vi "SRS830_GetXY.vi"(8 "error in (no error)":errorcluster, 11 "SRS 830":refnum<visa-resource-name>) -> (0 "error out (no error)":errorcluster, 1 "Y":dbl, 2 "X":dbl, 3 "SRS 830 Out":refnum<visa-resource-name>)   [LabVIEW 2014]
uses:
  Stanford Research 830/Stanford Research 830.lvlib
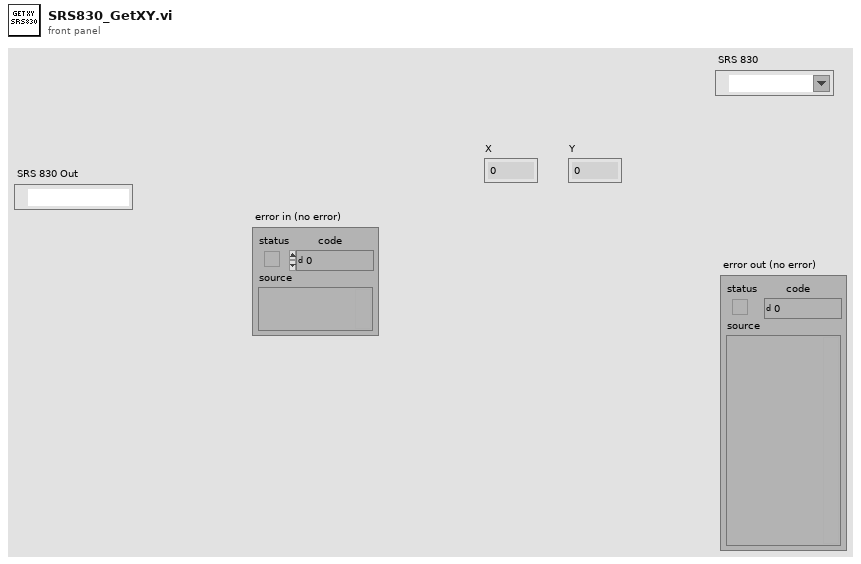
[diagram p1: front panel]
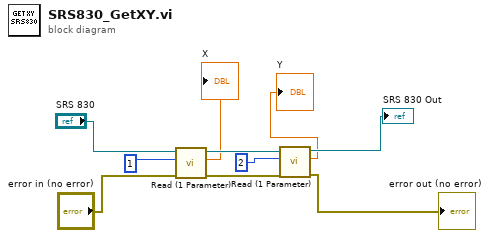
[diagram p0: block diagram]
diagram:
  n1 = call "Read (1 Parameter).vi"("error in (no error)"="error in (no error)", "Parameter (1: X)"=1, "VISA resource name"="SRS 830") -> ("error out"=w9:errorcluster, "Measurement"=→"X":dbl, "VISA resource name out"=w6:refnum<visa-resource-name>)  [unwired: 6 in]
  n2 = call "Read (1 Parameter).vi"("error in (no error)"=w9, "Parameter (1: X)"=2, "VISA resource name"=w6) -> ("error out"=→"error out (no error)":errorcluster, "Measurement"=→"Y":dbl, "VISA resource name out"=→"SRS 830 Out":refnum<visa-resource-name>)  [unwired: 6 in]
